vi "Actor Destroy.vi"(11 "Process in":refnum<class "ABD.lvclass">) -> (0 "error out":errorcluster, 3 "Process out":refnum<class "ABD.lvclass">)   [LabVIEW 2021, in "ABD.lvlib" / "ABD.lvclass"]
uses:
  ABD.lvclass
  ABD.lvclass/ABD.ctl
  LVCAM/LVCAM/Actor/Actor.lvclass
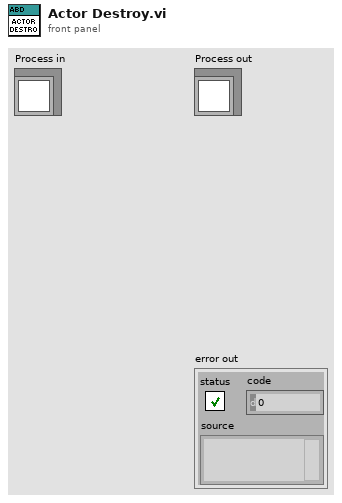
[diagram p1: front panel]
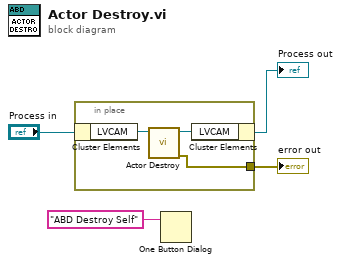
[diagram p0: block diagram]
diagram:
  n1 = in-place {
    in-place-border: [w5] -> w4
    n2 = in-place-cluster #1("Process in") -> ("LVCAM"=w7:refnum<class "Actor.lvclass">)
    n3 = call-dynamic "Actor Destroy.vi"("Actor Destroy in"=w7) -> ("error out"=w5:errorcluster, "Actor Destroy out"=w6:refnum<class "Actor.lvclass">)  [unwired: 9 in]
    n4 = in-place-cluster #1("LVCAM"=w6) -> (→"Process out":refnum<class "ABD.lvclass">)
  }
  "error out" <- w4
  n5 = One Button Dialog(message="ABD Destroy Self") -> ()  [unwired: 1 in, 1 out]
